vi "WPI_InterruptClose.vi"(8 "error in (no error)":errorcluster, 10 "Close Dependencies":bool=TRUE, 11 "InterruptRef":T1={"DevStatus"={"status"=FALSE, "code"=0, "source"=""}, "InterruptIndex"=enum."Invalid"}) -> (0 "error out":errorcluster)   [LabVIEW 2017]
doc: "Closes the reference to the interrupt you specify. Use this VI to close each interrupt reference that you open with the Open VI.\n\nThis software is licensed. Open the labview\\readme\\WPI Robotics Library Open Source License.txt file for more information."
uses:
  <vilib>/Rock Robotics/WPI/Interrupt/WPI_InterruptRef.ctl
  <vilib>/Rock Robotics/SystemInterfaces/Interrupt/FPGA_InterruptIndex.ctl
  <vilib>/Rock Robotics/WPI/Interrupt/WPI_InterruptCacheOp.ctl
  <vilib>/Rock Robotics/SystemInterfaces/CounterEncoderSourceConvertion/FPGA_CounterEncoderSourceConvertionLVSourceType.ctl
  <vilib>/Rock Robotics/SystemInterfaces/DIO/FPGA_DIODigitalSourceChannel.ctl
  <vilib>/Rock Robotics/SystemInterfaces/AnalogTrigger/FPGA_AnalogTriggerIndex.ctl
  <vilib>/Rock Robotics/SystemInterfaces/AnalogTrigger/FPGA_AnalogTriggerOutType.ctl
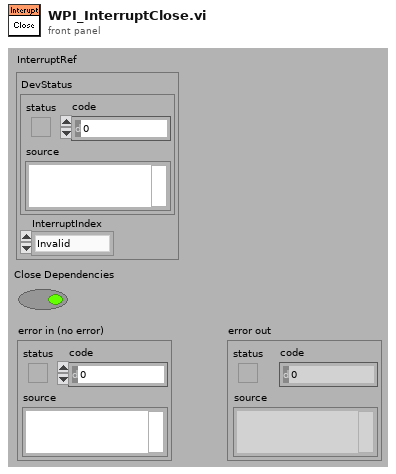
[diagram p1: front panel]
types:
  T1 = typedef "WPI_InterruptRef.ctl" = cluster{"DevStatus":errorcluster, "InterruptIndex":T2}
  T2 = typedef "FPGA_InterruptIndex.ctl" = enum8{"0", "1", "2", "3", "4", "5", "6", "7", "Invalid"}
  T3 = typedef "FPGA_CounterEncoderSourceConvertionLVSourceType.ctl" = cluster{"DevStatus":errorcluster, "AnalogTriggerMode?":bool, "DigitalMode":cluster{"DIO Channel":T4}, "AnalogTriggerMode":cluster{"AnalogTriggerIndex":T5, "OutputType":T6}}
  T4 = typedef "FPGA_DIODigitalSourceChannel.ctl" = enum8{"DIO 0", "DIO 1", "DIO 2", "DIO 3", "DIO 4", "DIO 5", "DIO 6", "DIO 7", "DIO 8", "DIO 9", "DIO MXP 0", "DIO MXP 1", "DIO MXP 2", "DIO MXP 3", "DIO MXP 4", "DIO MXP 5", "DIO MXP 6", "DIO MXP 7", "DIO MXP 8", "DIO MXP 9", "DIO MXP 10", "DIO MXP 11", "DIO MXP 12", "DIO MXP 13", "DIO MXP 14", "DIO MXP 15", "Disabled"}
  T5 = typedef "FPGA_AnalogTriggerIndex.ctl" = enum8{"Trig 0", "Trig 1", "Trig 2", "Trig 3", "Trig 4", "Trig 5", "Trig 6", "Trig 7", "Invalid"}
  T6 = typedef "FPGA_AnalogTriggerOutType.ctl" = enum16{"InWindow", "TriggerState", "Rising", "Falling"}
  T7 = typedef "WPI_InterruptCacheOp.ctl" = enum16{"Acquire", "Release"}
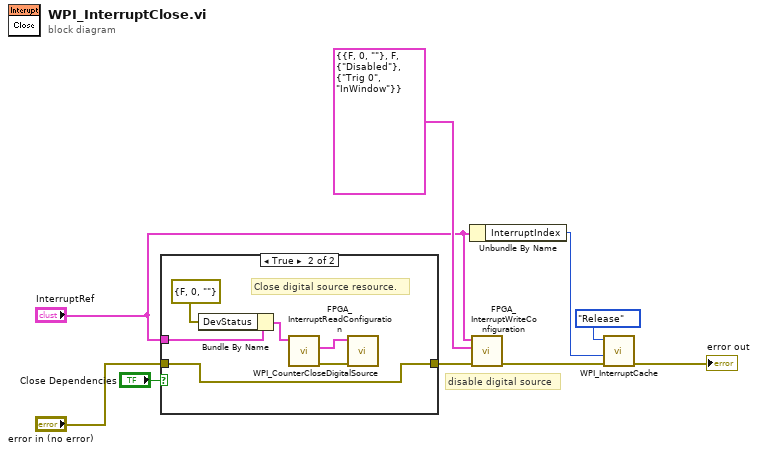
[diagram p0: block diagram]
diagram:
  # "disable digital source"
  n1 = case shown="True" "Close Dependencies" {
    tunnel: "InterruptRef" -> [_ w14]
    tunnel: [w10 w12] -> w5
    tunnel: "error in (no error)" -> [w10 w12]
    frame False {
    }
    frame True {
      # "Close digital source resource."
      n2 = Bundle By Name(cluster=w14, "DevStatus"=errorcluster {"status"=FALSE, "code"=0, "source"=""}) -> (w13:T1)
      n3 = call <vilib>:"FPGA_InterruptReadConfiguration.vi"("InteruptRef in"=w13) -> ("error out"=w15:errorcluster, "Source"=w16:T3)  [unwired: 1 in, 8 out]
      n4 = call <vilib>:"WPI_CounterCloseDigitalSource.vi"("error in"=w15, "UpSource"=w16) -> ()  [unwired: 6 out]
    }
  }
  n5 = Unbundle By Name("InterruptRef") -> ("InterruptIndex"=w9:T2)
  n6 = call <vilib>:"FPGA_InterruptWriteConfiguration.vi"("error in (no error)"=w5, "Source"=T3 {"DevStatus"={"status"=FALSE, "code"=0, "source"=""}, "AnalogTriggerMode?"=FALSE, "DigitalMode"={"DIO Channel"=enum."Disabled"}, "AnalogTriggerMode"={"AnalogTriggerIndex"=enum."Trig 0", "OutputType"=enum."InWindow"}}, "InteruptRef in"="InterruptRef") -> ("error out"=w4:errorcluster)  [unwired: 3 in, 5 out]
  n7 = call <vilib>:"WPI_InterruptCache.vi"("error in (no error)"=w4, "InterruptIndexToRelease"=w9, "InterruptCacheOp"=WPI_InterruptCacheOp."Release") -> ("error out"=→"error out":errorcluster)  [unwired: 8 out]
